vi "CPU_Quadrature_DDS_CDB.vi"(7 "reset":bool, 9 "Freq Offset":dbl=-21389.0, 11 "size":i32) -> (3 "T1D_CSG out":cdb[](array[numeric]) format="%.3f", 4 "dt":dbl)   [LabVIEW 2020]
uses:
  <vilib>/Analysis/NI_AALBase.lvlib
panel:
  in  "phase(degrees)":dbl format="%0.2f"
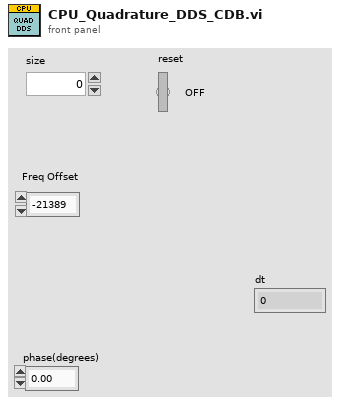
[diagram p1: front panel]
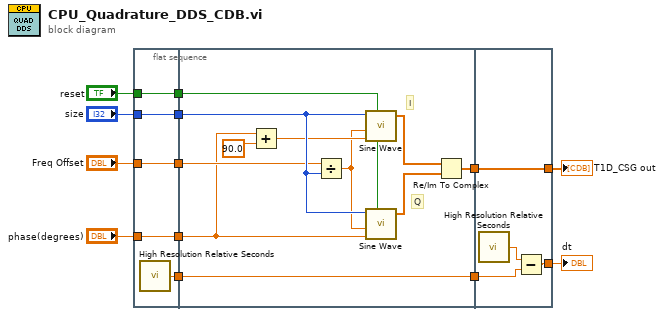
[diagram p0: block diagram]
diagram:
  n1 = flat-sequence {
    tunnel: "size" -> [w17]
    tunnel: "Freq Offset" -> [w18]
    tunnel: [w18] -> w13
    tunnel: [w17] -> w12
    tunnel: [w16] -> w11
    tunnel: [w15] -> w6
    tunnel: "reset" -> [w15]
    tunnel: [w14] -> w4
    tunnel: "phase(degrees)" -> [w14]
    tunnel: w13 -> [w23]
    tunnel: w12 -> [w24]
    tunnel: [w29] -> w10
    tunnel: w11 -> [w29]
    tunnel: w6 -> [w25]
    tunnel: w4 -> [w22]
    tunnel: [w26] -> w2
    tunnel: w10 -> [w32]
    tunnel: [w31] -> w7
    tunnel: [w30] -> w1
    tunnel: w2 -> [w30]
    frame #0 {
      n2 = call <vilib>:"High Resolution Relative Seconds.vi"() -> ("relative seconds"=w16:dbl)
    }
    frame #1 {
      # "Q"
      # "I"
      n3 = Add(x=w22, y=90.0) -> (x+y=w21:dbl)
      n4 = Divide(x=w23, y=w24) -> (x/y=w19:dbl)
      n5 = call <vilib>:"Sine Wave.vi"("samples"=w24, "frequency"=w19, "phase in"=w21, "reset phase"=w25) -> ("sine wave"=w28:dbl[])  [unwired: 1 in, 2 out]
      n6 = call <vilib>:"Sine Wave.vi"("samples"=w24, "frequency"=w19, "phase in"=w22, "reset phase"=w25) -> ("sine wave"=w27:dbl[])  [unwired: 1 in, 2 out]
      n7 = Re/Im To Complex(1:w27, 2:w28) -> (0:w26:cdb[])
    }
    frame #2 {
      n8 = call <vilib>:"High Resolution Relative Seconds.vi"() -> ("relative seconds"=w33:dbl)
      n9 = Subtract(x=w33, y=w32) -> (x-y=w31:dbl)
    }
  }
  "T1D_CSG out" <- w1
  "dt" <- w7
